vi "pneumatics.vi"(0 "Clear PCM Sticky Faults":bool caption="Clear PDP Sticky Faults:\nThis resets the faults on the PDP and \nthe associated LEDs. These faults do \nnot clear with a robot reboot.") -> (1 "Full":bool, 2 "Charging":bool, 3 "On/Off":bool=TRUE)   [LabVIEW 2015]
uses:
  <vilib>/Rock Robotics/Network Tables/NT Read Boolean Array.vi
  <vilib>/Rock Robotics/Network Tables/NT Write Boolean.vi
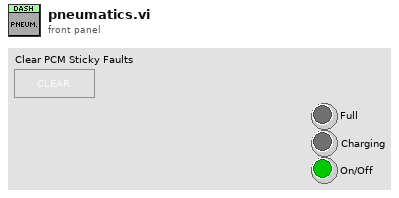
[diagram p1: front panel]
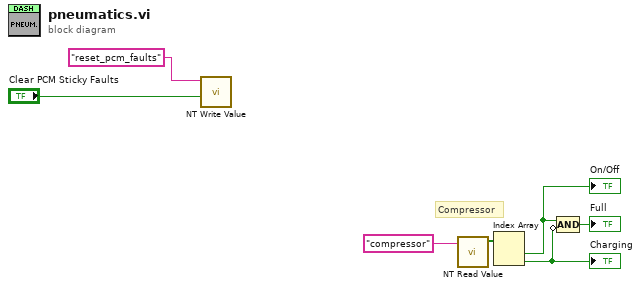
[diagram p0: block diagram]
diagram:
  # "Compressor"
  n1 = call-poly <vilib>:"NT Write Value.vi"("Boolean"="Clear PCM Sticky Faults", "Name"="reset_pcm_faults") -> ()  [unwired: 9 in, 1 out]
  n2 = call-poly <vilib>:"NT Read Value.vi"("Name"="compressor") -> ("Boolean Array"=w3:bool[])  [unwired: 9 in, 1 out]
  n3 = Index Array(array=w3) -> (element #1=w5:bool, element #2=w4:bool)  [unwired: 2 in]
  "Charging" <- w4
  "On/Off" <- w5
  n4 = Compound Arithmetic op=AND(w5, invert w4) -> (→"Full":bool)
